vi "CAL_GCP_L.vi"(9 "출력 클러스터 2":T1, 10 "B_ACC":sgl, 11 "L_ROLL":sgl) -> (0 "L_Period":sgl, 1 "L_GCP":sgl, 2 "L_Ctrl_Start":bool, 3 "L_NUM":u32, 4 "L_Run_OK":bool)   [LabVIEW 2019]
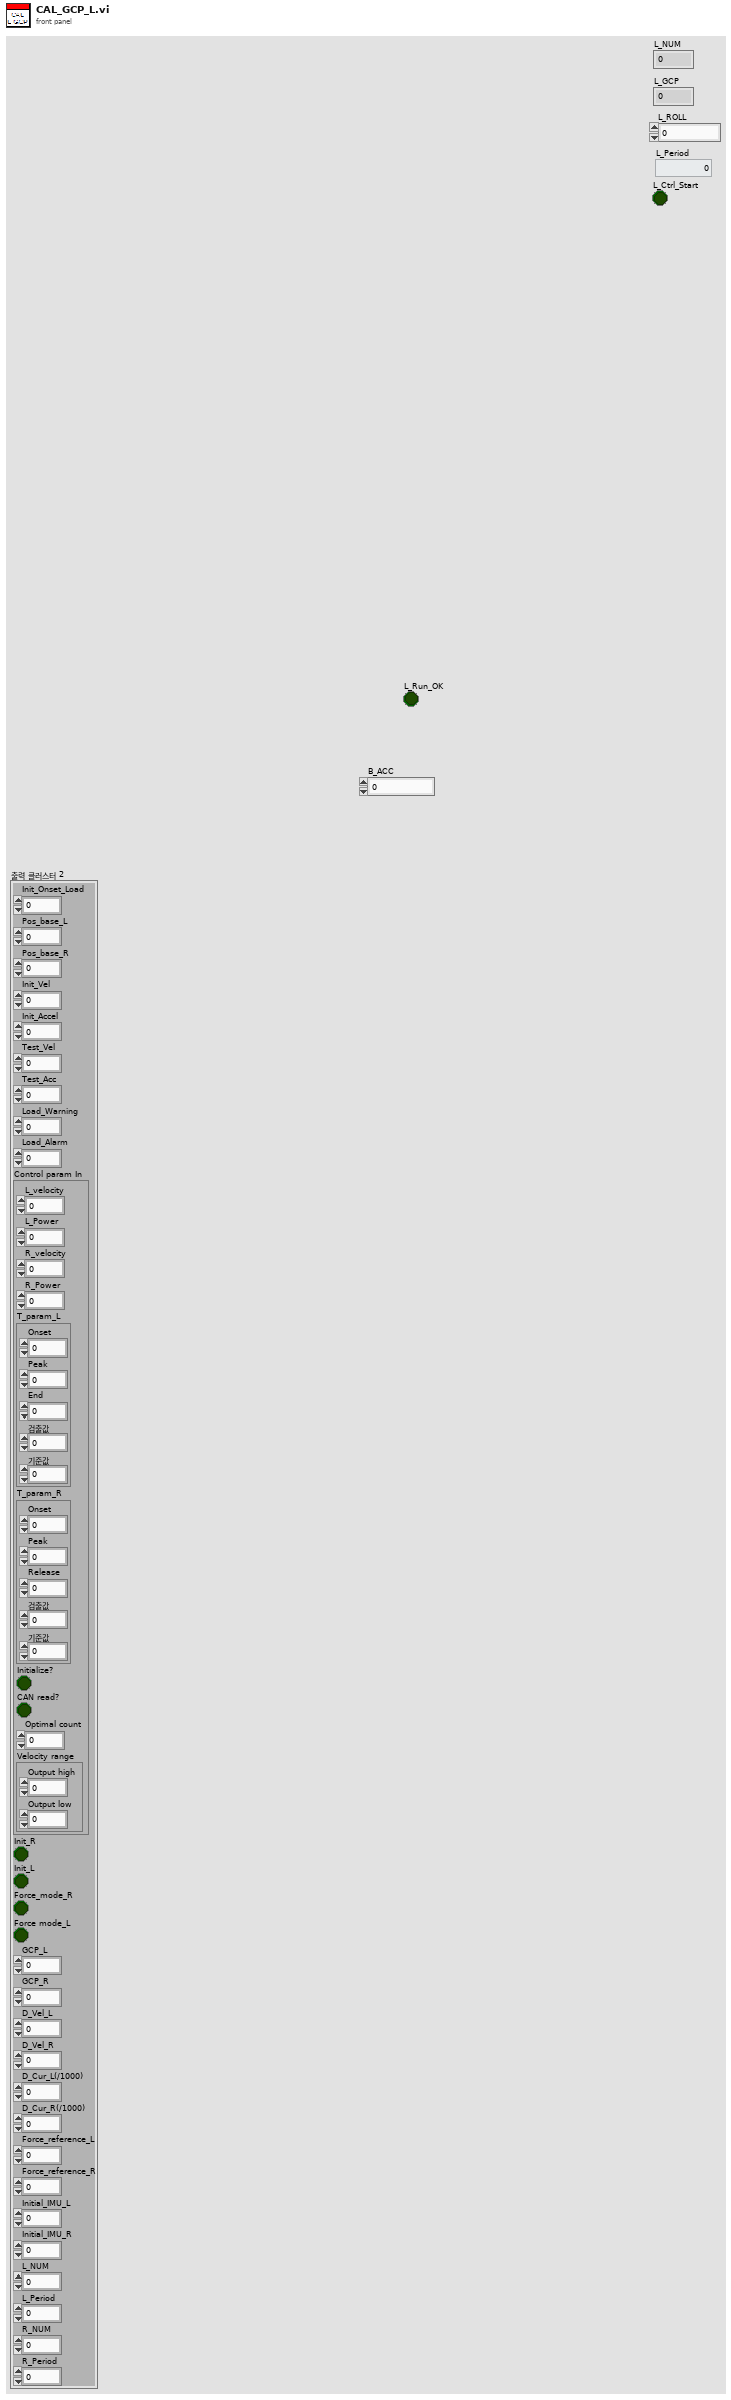
[diagram p1: front panel]
types:
  T1 = cluster{"Init_Onset_Load":sgl, "Pos_base_L":sgl, "Pos_base_R":sgl, "Init_Vel":i32, "Init_Accel":u32, "Test_Vel":i32, "Test_Acc":u32, "Load_Warning":sgl, "Load_Alarm":sgl, "Control param In":cluster{"L_velocity":u32, "L_Power":sgl, "R_velocity":u32, "R_Power":sgl, "T_param_L":cluster{"Onset":sgl, "Peak":sgl, "End":sgl, "검출값":sgl, "기준값":sgl}, "T_param_R":cluster{"Onset":sgl, "Peak":sgl, "Release":sgl, "검출값":sgl, "기준값":sgl}, "Initialize?":bool, "CAN read?":bool, "Optimal count":i32, "Velocity range":cluster{"Output high":dbl, "Output low":dbl}}, "Init_R":bool, "Init_L":bool, "Force_mode_R":bool, "Force mode_L":bool, "GCP_L":sgl, "GCP_R":sgl, "D_Vel_L":sgl, "D_Vel_R":sgl, "D_Cur_L(/1000)":sgl, "D_Cur_R(/1000)":sgl, "Force_reference_L":sgl, "Force_reference_R":sgl, "Initial_IMU_L":sgl, "Initial_IMU_R":sgl, "L_NUM":u32, "L_Period":i16, "R_NUM":u32, "R_Period":i16}
  T2 = enum16{"Init", "HF", "Cross", "HE", "Cross_E", "Init_F"}
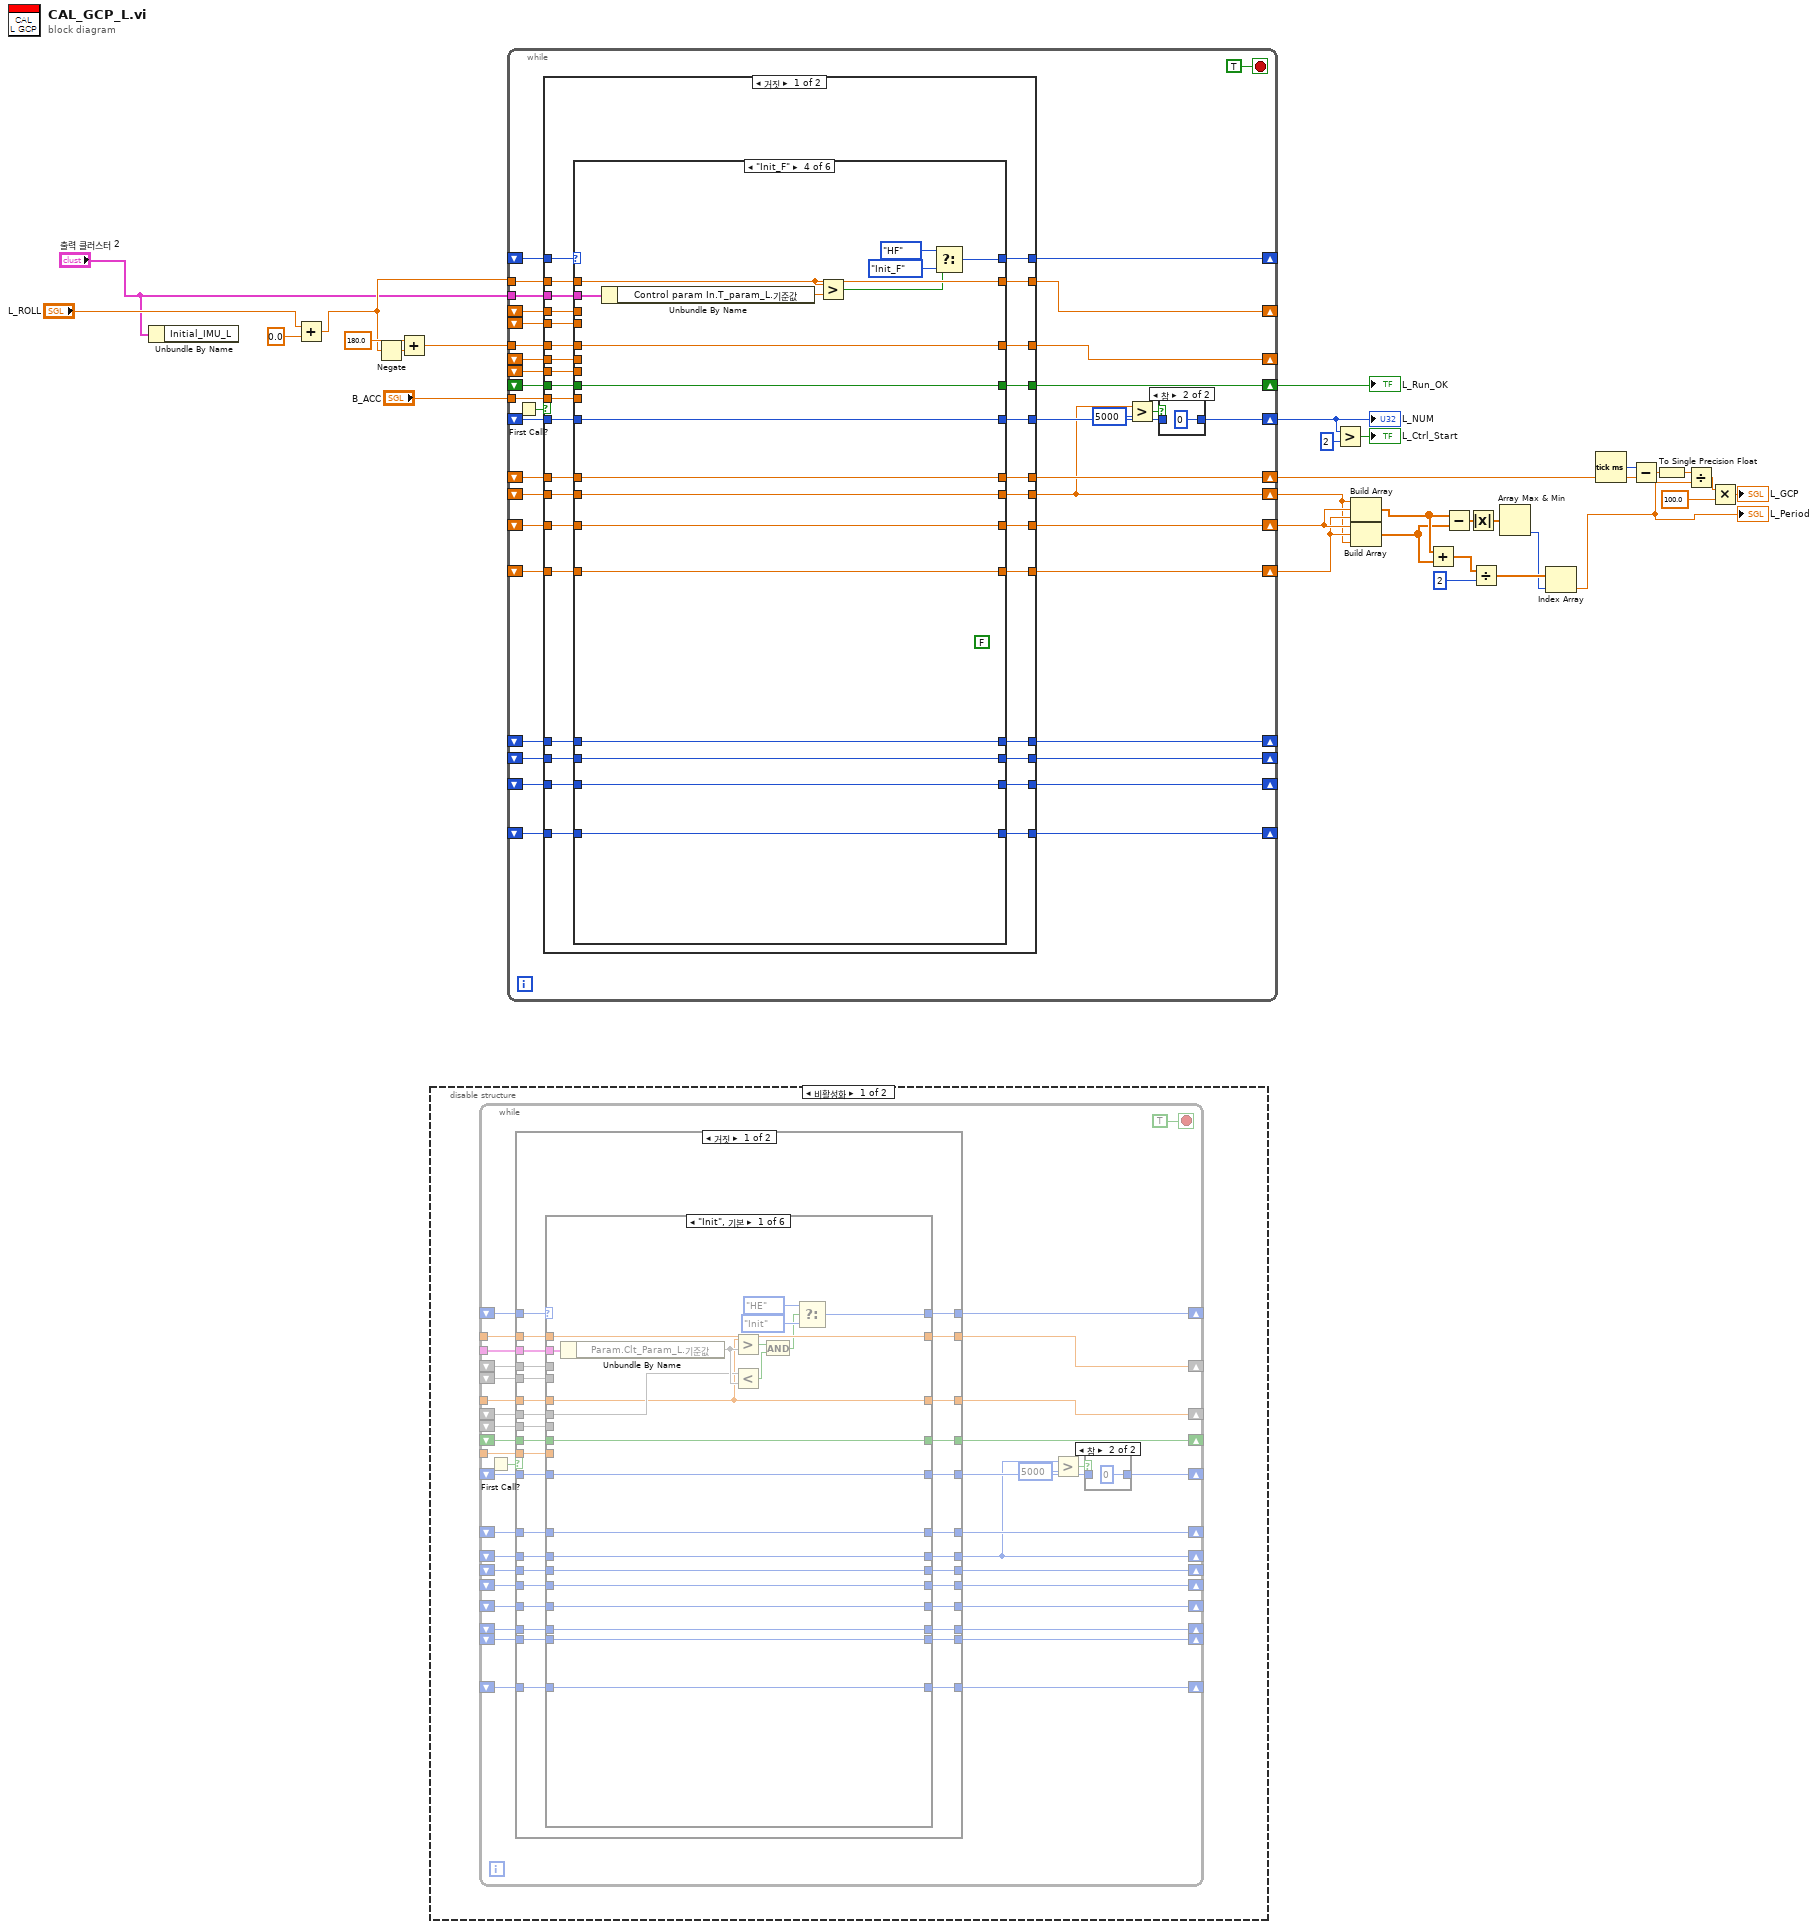
[diagram p0: block diagram]
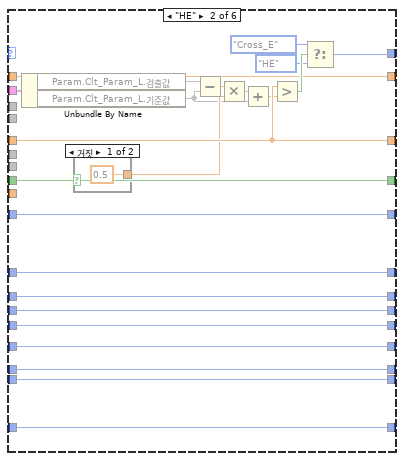
[diagram p2: hidden frame]
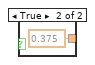
[diagram p3: hidden frame]
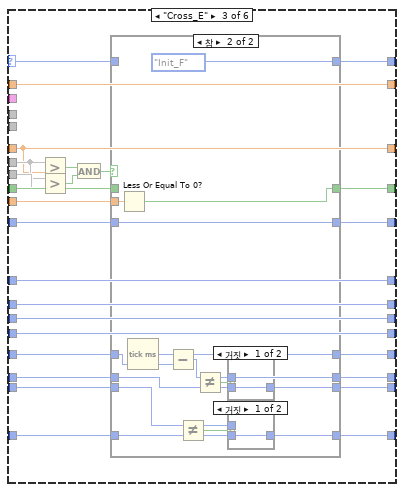
[diagram p4: hidden frame]
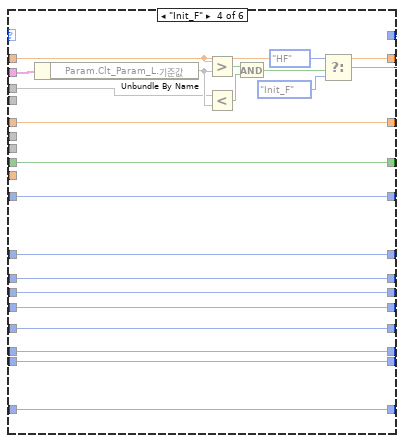
[diagram p8: hidden frame]
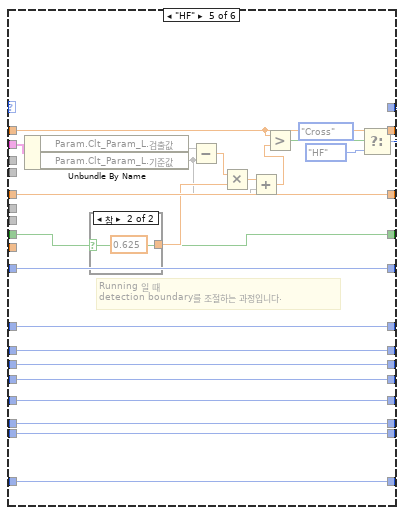
[diagram p9: hidden frame]
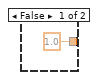
[diagram p10: hidden frame]
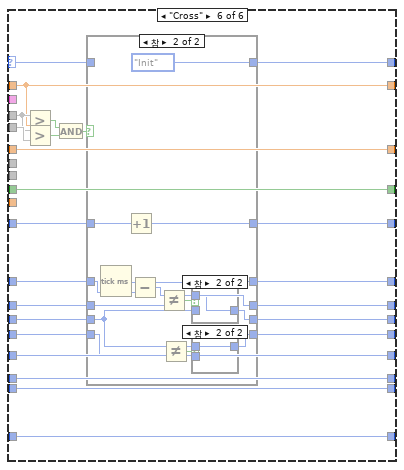
[diagram p11: hidden frame]
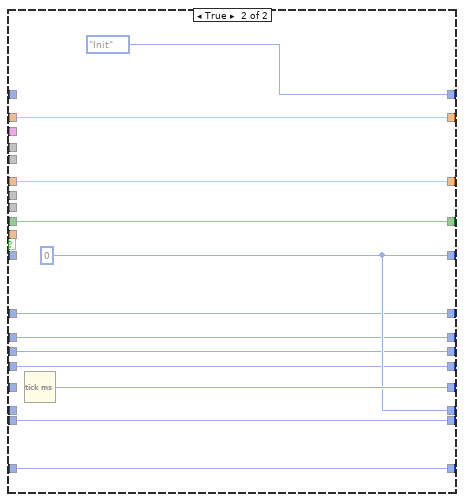
[diagram p15: hidden frame]
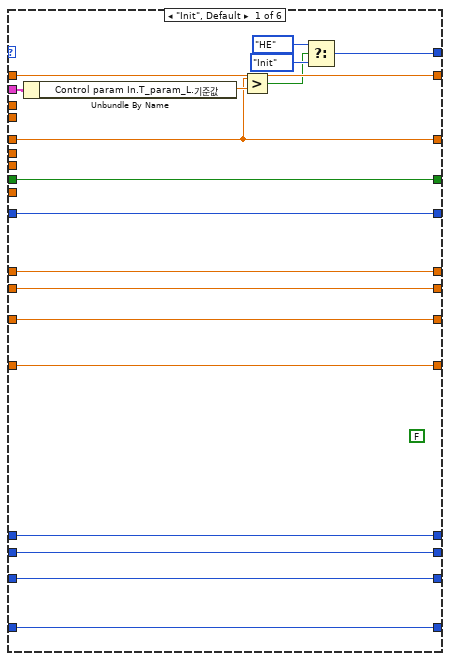
[diagram p18: hidden frame]
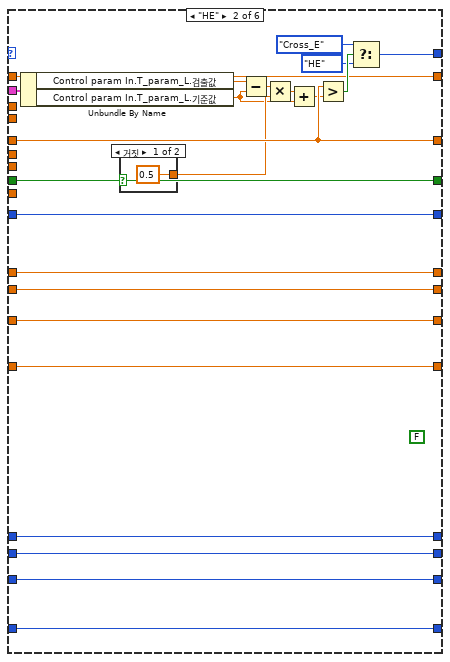
[diagram p19: hidden frame]
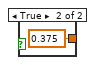
[diagram p20: hidden frame]
diagram:
  n1 = Unbundle By Name("출력 클러스터 2") -> ()  [unwired: 1 out]
  n2 = Add(x="L_ROLL", y=sgl 0.0) -> (x+y=w4:sgl)
  n3 = Negate(x=w4) -> (-x=w22:sgl)
  n4 = Add(x=sgl 180.0, y=w22) -> (x+y=w21:sgl)
  n5 = disable-structure shown="비활성화" {
    frame Disabled {
      n6 = while {
        tunnel: _ -> [w65]
        tunnel: _ -> [w62]
        shift-right: [w34] -> _
        shift-left: _ -> [w33]
        shift-right: [w66] -> _
        shift-left: _ -> [w61]
        shift-left: _ -> [w60]
        shift-right: [w57] -> _
        shift-left: _ -> [w64]
        shift-right: [w47] -> _
        shift-left: _ -> [w63]
        tunnel: _ -> [w55]
        shift-right: [w54] -> _
        shift-left: _ -> [w53]
        shift-left: _ -> [w52]
        shift-right: [w51] -> _
        shift-left: _ -> [w50]
        tunnel: _ -> [w49]
        shift-right: [w46] -> _
        shift-left: _ -> [w48]
        shift-right: [w39] -> _
        shift-left: _ -> [w38]
        shift-right: [w36] -> _
        shift-left: _ -> [w37]
        shift-right: [w45] -> _
        shift-left: _ -> [w44]
        shift-right: [w42] -> _
        shift-left: _ -> [w43]
        shift-right: [w41] -> _
        shift-left: _ -> [w40]
        shift-right: [w32] -> _
        shift-left: _ -> [w35]
        stop <- TRUE stop-if-true
        n7 = First Call?() -> (First Call?: T/F=w67:bool)
        n8 = case shown="거짓" w67 {
          tunnel: [w98 w302] -> w66
          tunnel: w65 -> [w99 w302]
          tunnel: w64 -> [w96 _]
          tunnel: [w97 w300] -> w56
          tunnel: [w94 w301] -> w47
          tunnel: [w93 w300] -> w46
          tunnel: w63 -> [w95 _]
          tunnel: w62 -> [w100 _]
          tunnel: w61 -> [w92 _]
          tunnel: w60 -> [w91 _]
          tunnel: w55 -> [w90 w299]
          tunnel: [w89 w299] -> w54
          tunnel: w53 -> [w88 _]
          tunnel: w52 -> [w87 _]
          tunnel: [w85 w298] -> w51
          tunnel: w50 -> [w86 w298]
          tunnel: w49 -> [w84 _]
          tunnel: w48 -> [w83 _]
          tunnel: [w82 w297] -> w45
          tunnel: w44 -> [w81 w297]
          tunnel: w43 -> [w80 w296]
          tunnel: [w79 w296] -> w42
          tunnel: [w78 w295] -> w41
          tunnel: w40 -> [w77 w295]
          tunnel: [w76 w294] -> w39
          tunnel: w38 -> [w75 w294]
          tunnel: w37 -> [w74 w293]
          tunnel: [w73 w293] -> w36
          tunnel: [w72 w292] -> w32
          tunnel: w35 -> [w71 w292]
          tunnel: [w69 T2."Init"] -> w34
          tunnel: w33 -> [w70 _]
          frame False {
            n9 = case shown="\"Init\", 기본" w70 {
              selector: w70 -> [_ _ w172 _ _ w267]
              tunnel: w100 -> [w118 w136 _ w212 w241 _]
              tunnel: w99 -> [w117 w143 w152 w209 w239 w260]
              tunnel: [w117 w143 w152 w209 w239 w260] -> w98
              tunnel: [w116 w142 w170 w206 w238 w262] -> w97
              tunnel: w96 -> [w116 w142 w171 w206 w238 w263]
              tunnel: w95 -> [w115 w141 w168 w205 w237 w255]
              tunnel: [w115 w141 w169 w205 w237 w255] -> w94
              tunnel: [w111 w140 w167 w204 w236 w258] -> w93
              tunnel: w92 -> [_ _ _ w211 _ w261]
              tunnel: w91 -> [_ _ _ _ _ w266]
              tunnel: w90 -> [w113 w135 w151 w208 w232 w252]
              tunnel: [w113 w135 w151 w208 w232 w252] -> w89
              tunnel: w88 -> [w114 _ w159 _ _ _]
              tunnel: w87 -> [_ _ w160 _ _ _]
              tunnel: w86 -> [w112 w126 w166 w207 w226 w251]
              tunnel: [w112 w126 w165 w207 w226 w251] -> w85
              tunnel: w84 -> [_ _ w164 _ _ _]
              tunnel: w83 -> [w111 w140 w158 w204 w236 w258]
              tunnel: [w110 w139 w157 w202 w235 w257] -> w82
              tunnel: w81 -> [w110 w139 w156 w202 w235 w257]
              tunnel: w80 -> [w109 w138 w155 w201 w234 w256]
              tunnel: [w109 w138 w154 w201 w234 w256] -> w79
              tunnel: [w108 w137 w153 w203 w233 w254] -> w78
              tunnel: w77 -> [w108 w137 w153 w203 w233 w253]
              tunnel: [w107 w134 w149 w199 w231 w250] -> w76
              tunnel: w75 -> [w107 w134 w149 w199 w231 w249]
              tunnel: w74 -> [w106 w133 w150 w198 w230 w248]
              tunnel: [w106 w133 w150 w198 w230 w247] -> w73
              tunnel: [w105 w125 w148 w200 w222 w246] -> w72
              tunnel: w71 -> [w105 w125 w148 w200 w222 w245]
              tunnel: [w104 w122 w147 w210 w219 w244] -> w69
              frame "Init", Default {
                n10 = Unbundle By Name(w118) -> ("Param.Clt_Param_L.기준값"=w119)
                n11 = Greater?(x=w113, y=w119) -> (0:w121:bool)
                n12 = Less?(x=w114, y=w119) -> (x < y?=w120:bool)
                n13 = And(x=w121, y=w120) -> (x .and. y?=w102:bool)
                n14 = Select(t=T2."HE", s=w102, f=T2."Init") -> (s? t:f=w104:T2)
              }
              frame "HE" {
                n15 = Unbundle By Name(w136) -> ("Param.Clt_Param_L.검출값"=w131, "Param.Clt_Param_L.기준값"=w128)
                n16 = case shown="거짓" w126 {
                  tunnel: [sgl 0.5 ("y") sgl 0.375 ("y")] -> w132
                  frame False {
                  }
                  frame True {
                  }
                }
                n17 = Subtract(x=w131, y=w128) -> (x-y=w130:dbl)
                n18 = Multiply(x=w130, y=w132) -> (x*y=w129:sgl)
                n19 = Add(x=w129, y=w128) -> (x+y=w127:sgl)
                n20 = Greater?(x=w135, y=w127) -> (0:w144:bool)
                n21 = Select(t=T2."Cross_E", s=w144, f=T2."HE") -> (s? t:f=w122:T2)
              }
              frame "Cross_E" {
                n22 = Greater?(x=w159, y=w151) -> (0:w162:bool)
                n23 = Greater?(x=w159, y=w160) -> (0:w163:bool)
                n24 = And(x=w162, y=w163) -> (x .and. y?=w161:bool)
                n25 = case shown="참" w161 {
                  tunnel: w172 -> [w177 _]
                  tunnel: [w177 T2."Init_F"] -> w147
                  tunnel: w171 -> [w178 w181]
                  tunnel: [w178 w181] -> w170
                  tunnel: w168 -> [w179 w193]
                  tunnel: [w175 w180] -> w167
                  tunnel: [w179 w192] -> w169
                  tunnel: w166 -> [w176 _]
                  tunnel: [w176 w188] -> w165
                  tunnel: w164 -> [_ w189]
                  tunnel: w158 -> [w175 w187]
                  tunnel: [w174 w186] -> w157
                  tunnel: w156 -> [w174 w185]
                  tunnel: w155 -> [w173 w184]
                  tunnel: [w173 w183] -> w154
                  frame False {
                  }
                  frame True {
                    n26 = Less Or Equal To 0?(x=w189) -> (x <= 0?=w188:bool)
                    n27 = Tick Count (ms)() -> (millisecond timer value=w192:u32)
                    n28 = Subtract(x=w192, y=w193) -> (x-y=w180:u32)
                    n29 = Not Equal?(x=w185, y=w184) -> (x != y?=w190:bool)
                    n30 = Not Equal?(x=w180, y=w187) -> (x != y?=w191:bool)
                    n31 = case shown="거짓" w191 {
                      tunnel: [w196 w197] -> w186
                      tunnel: w180 -> [_ w197]
                      tunnel: w187 -> [w196 _]
                      frame False {
                      }
                      frame True {
                      }
                    }
                    n32 = case shown="거짓" w190 {
                      tunnel: w185 -> [_ w195]
                      tunnel: w184 -> [w194 _]
                      tunnel: [w194 w195] -> w183
                      frame False {
                      }
                      frame True {
                      }
                    }
                  }
                }
              }
              frame "Init_F" {
                n33 = Unbundle By Name(w212) -> ("Param.Clt_Param_L.기준값"=w216)
                n34 = Greater?(x=w209, y=w216) -> (0:w218:bool)
                n35 = Less?(x=w211, y=w216) -> (x < y?=w217:bool)
                n36 = And(x=w218, y=w217) -> (x .and. y?=w214:bool)
                n37 = Select(t=T2."HF", s=w214, f=T2."Init_F") -> (s? t:f=w210:T2)
              }
              frame "HF" {
                # "Running 일 때 \ndetection boundary를 조절하는 과정입니다."
                n38 = Unbundle By Name(w241) -> ("Param.Clt_Param_L.검출값"=w229, "Param.Clt_Param_L.기준값"=w224)
                n39 = case shown="참" w226 {
                  tunnel: [sgl 1.0 ("y") sgl 0.625 ("y")] -> w227
                  frame False {
                  }
                  frame True {
                  }
                }
                n40 = Subtract(x=w229, y=w224) -> (x-y=w228:dbl)
                n41 = Multiply(x=w228, y=w227) -> (x*y=w225:sgl)
                n42 = Add(x=w225, y=w224) -> (x+y=w223:sgl)
                n43 = Greater?(x=w239, y=w223) -> (0:w240:bool)
                n44 = Select(t=T2."Cross", s=w240, f=T2."HF") -> (s? t:f=w219:T2)
              }
              frame "Cross" {
                n45 = Greater?(x=w261, y=w260) -> (0:w259:bool)
                n46 = Greater?(x=w261, y=w266) -> (0:w265:bool)
                n47 = And(x=w259, y=w265) -> (x .and. y?=w264:bool)
                n48 = case shown="참" w264 {
                  tunnel: w267 -> [w272 _]
                  tunnel: [w272 T2."Init"] -> w244
                  tunnel: w263 -> [w273 w276]
                  tunnel: [w273 w275] -> w262
                  tunnel: [w271 w283] -> w254
                  tunnel: w253 -> [w271 w284]
                  tunnel: [w270 w282] -> w250
                  tunnel: w249 -> [w270 w281]
                  tunnel: w248 -> [w269 w280]
                  tunnel: [w269 w279] -> w247
                  tunnel: [w268 w274] -> w246
                  tunnel: w245 -> [w268 w278]
                  frame False {
                  }
                  frame True {
                    n49 = Tick Count (ms)() -> (millisecond timer value=w283:u32)
                    n50 = Increment(x=w276) -> (x+1=w275:u32)
                    n51 = Subtract(x=w283, y=w284) -> (x-y=w274:u32)
                    n52 = Not Equal?(x=w274, y=w278) -> (x != y?=w286:bool)
                    n53 = Not Equal?(x=w281, y=w280) -> (x != y?=w285:bool)
                    n54 = case shown="참" w286 {
                      tunnel: w274 -> [_ w290]
                      tunnel: [w289 w290] -> w282
                      tunnel: w281 -> [w289 _]
                      frame False {
                      }
                      frame True {
                      }
                    }
                    n55 = case shown="참" w285 {
                      tunnel: w281 -> [_ w288]
                      tunnel: w280 -> [w287 _]
                      tunnel: [w287 w288] -> w279
                      frame False {
                      }
                      frame True {
                      }
                    }
                  }
                }
              }
            }
          }
          frame True {
            w300 = u32 0
            n56 = Tick Count (ms)() -> (millisecond timer value=w301:u32)
          }
        }
        n57 = Greater?(x=w32, y=u32 5000) -> (0:w58:bool)
        n58 = case shown="참" w58 {
          tunnel: [w303 u32 0] -> w57
          tunnel: w56 -> [w303 _]
          frame False {
          }
          frame True {
          }
        }
      }
    }
    frame Enabled {
    }
  }
  n59 = while {
    tunnel: w4 -> [w338]
    tunnel: "출력 클러스터 2" -> [w335]
    shift-right: [w307] -> _
    shift-left: _ -> [w306]
    shift-right: [w339] -> _
    shift-left: _ -> [w334]
    shift-left: _ -> [w333]
    shift-right: [w330] -> w18
    shift-left: _ -> [w337]
    shift-right: [w320] -> _
    shift-left: _ -> [w336]
    tunnel: w21 -> [w328]
    shift-right: [w327] -> _
    shift-left: _ -> [w326]
    shift-left: _ -> [w325]
    shift-right: [w324] -> w19
    shift-left: _ -> [w323]
    tunnel: "B_ACC" -> [w322]
    shift-right: [w319] -> _
    shift-left: _ -> [w321]
    shift-right: [w312] -> w16
    shift-left: _ -> [w311]
    shift-right: [w309] -> w15
    shift-left: _ -> [w310]
    shift-right: [w318] -> _
    shift-left: _ -> [w317]
    shift-right: [w315] -> _
    shift-left: _ -> [w316]
    shift-right: [w314] -> w17
    shift-left: _ -> [w313]
    shift-right: [w305] -> w14
    shift-left: _ -> [w308]
    stop <- TRUE stop-if-true
    n60 = First Call?() -> (First Call?: T/F=w340:bool)
    n61 = case shown="거짓" w340 {
      tunnel: [w371 w571] -> w339
      tunnel: w338 -> [w372 w571]
      tunnel: w337 -> [w369 _]
      tunnel: [w370 w570] -> w329
      tunnel: [w367 w561] -> w320
      tunnel: [w366 w570] -> w319
      tunnel: w336 -> [w368 _]
      tunnel: w335 -> [w373 _]
      tunnel: w334 -> [w365 _]
      tunnel: w333 -> [w364 _]
      tunnel: w328 -> [w363 w569]
      tunnel: [w362 w569] -> w327
      tunnel: w326 -> [w361 _]
      tunnel: w325 -> [w360 _]
      tunnel: [w358 w568] -> w324
      tunnel: w323 -> [w359 w568]
      tunnel: w322 -> [w357 _]
      tunnel: w321 -> [w356 _]
      tunnel: [w355 w567] -> w318
      tunnel: w317 -> [w354 w567]
      tunnel: w316 -> [w353 w566]
      tunnel: [w352 w566] -> w315
      tunnel: [w351 w561] -> w314
      tunnel: w313 -> [w350 _]
      tunnel: [w349 w565] -> w312
      tunnel: w311 -> [w348 w565]
      tunnel: w310 -> [w347 w564]
      tunnel: [w346 w564] -> w309
      tunnel: [w345 w563] -> w305
      tunnel: w308 -> [w344 w563]
      tunnel: [w342 T2."Init"] -> w307
      tunnel: w306 -> [w343 _]
      frame False {
        n62 = case shown="\"Init_F\"" w343 {
          selector: w343 -> [_ _ w442 _ _ w536]
          tunnel: w373 -> [w390 w406 _ w484 w510 _]
          tunnel: w372 -> [w389 w413 w422 w482 w508 w529]
          tunnel: [w389 w413 w422 w482 w508 w529] -> w371
          tunnel: [w388 w412 w440 w479 w507 w531] -> w370
          tunnel: w369 -> [w388 w412 w441 w479 w507 w532]
          tunnel: w368 -> [w387 w411 w438 w478 w506 w524]
          tunnel: [w387 w411 w439 w478 w506 w524] -> w367
          tunnel: [w384 w410 w437 w477 w505 w527] -> w366
          tunnel: w365 -> [_ _ _ _ _ w530]
          tunnel: w364 -> [_ _ _ _ _ w535]
          tunnel: w363 -> [w386 w405 w421 w481 w501 w521]
          tunnel: [w386 w405 w421 w481 w501 w521] -> w362
          tunnel: w361 -> [_ _ w429 _ _ _]
          tunnel: w360 -> [_ _ w430 _ _ _]
          tunnel: w359 -> [w385 w396 w436 w480 w495 w520]
          tunnel: [w385 w396 w435 w480 w495 w520] -> w358
          tunnel: w357 -> [_ _ w434 _ _ _]
          tunnel: w356 -> [w384 w410 w428 w477 w505 w527]
          tunnel: [w383 w409 w427 w475 w504 w526] -> w355
          tunnel: w354 -> [w383 w409 w426 w475 w504 w526]
          tunnel: w353 -> [w382 w408 w425 w474 w503 w525]
          tunnel: [w382 w408 w424 w474 w503 w525] -> w352
          tunnel: [w381 w407 w423 w476 w502 w523] -> w351
          tunnel: w350 -> [w381 w407 w423 w476 w502 w522]
          tunnel: [w380 w404 w419 w472 w500 w519] -> w349
          tunnel: w348 -> [w380 w404 w419 w472 w500 w518]
          tunnel: w347 -> [w379 w403 w420 w471 w499 w517]
          tunnel: [w379 w403 w420 w471 w499 w516] -> w346
          tunnel: [w378 w395 w418 w473 w491 w515] -> w345
          tunnel: w344 -> [w378 w395 w418 w473 w491 w514]
          tunnel: [w377 w392 w417 w483 w488 w513] -> w342
          frame "Init", Default {
            (unwired) FALSE
            n63 = Unbundle By Name(w390) -> ("Control param In.T_param_L.기준값"=w391:sgl)
            n64 = Greater?(x=w386, y=w391) -> (0:w374:bool)
            n65 = Select(t=T2."HE", s=w374, f=T2."Init") -> (s? t:f=w377:T2)
          }
          frame "HE" {
            (unwired) FALSE
            n66 = Unbundle By Name(w406) -> ("Control param In.T_param_L.검출값"=w401:sgl, "Control param In.T_param_L.기준값"=w398:sgl)
            n67 = case shown="거짓" w396 {
              tunnel: [sgl 0.5 ("y") sgl 0.375 ("y")] -> w402
              frame False {
              }
              frame True {
              }
            }
            n68 = Subtract(x=w401, y=w398) -> (x-y=w400:sgl)
            n69 = Multiply(x=w400, y=w402) -> (x*y=w399:sgl)
            n70 = Add(x=w399, y=w398) -> (x+y=w397:sgl)
            n71 = Greater?(x=w405, y=w397) -> (0:w414:bool)
            n72 = Select(t=T2."Cross_E", s=w414, f=T2."HE") -> (s? t:f=w392:T2)
          }
          frame "Cross_E" {
            (unwired) FALSE
            n73 = Greater?(x=w429, y=w421) -> (0:w432:bool)
            n74 = Greater Or Equal?(x=w429, y=w430) -> (x >= y?=w433:bool)
            n75 = And(x=w432, y=w433) -> (x .and. y?=w431:bool)
            n76 = case shown="참" w431 {
              tunnel: w442 -> [w447 _]
              tunnel: [w447 T2."Init_F"] -> w417
              tunnel: w441 -> [w448 w456]
              tunnel: [w448 w456] -> w440
              tunnel: w438 -> [w449 w465]
              tunnel: [w445 w455] -> w437
              tunnel: [w449 w464] -> w439
              tunnel: w436 -> [w446 _]
              tunnel: [w446 w461] -> w435
              tunnel: w434 -> [_ w452]
              tunnel: w428 -> [w445 w454]
              tunnel: [w444 w460] -> w427
              tunnel: w426 -> [w444 w453]
              tunnel: w425 -> [w443 w459]
              tunnel: [w443 w458] -> w424
              frame False {
              }
              frame True {
                n77 = Tick Count (ms)() -> (millisecond timer value=w464:u32)
                n78 = Subtract(x=w464, y=w465) -> (x-y=w455:u32)
                n79 = Add(x=w452, y=9.8) -> (x+y=w450:dbl)
                n80 = Not Equal?(x=w453, y=w459) -> (x != y?=w462:bool)
                n81 = Not Equal?(x=w454, y=w453) -> (x != y?=w463:bool)
                n82 = Greater Or Equal To 0?(x=w450) -> (x >= 0?=w461:bool)
                n83 = case shown="거짓" w463 {
                  tunnel: [w468 w469] -> w460
                  tunnel: w454 -> [_ w469]
                  tunnel: w453 -> [w468 _]
                  frame False {
                  }
                  frame True {
                  }
                }
                n84 = case shown="거짓" w462 {
                  tunnel: w453 -> [_ w467]
                  tunnel: w459 -> [w466 _]
                  tunnel: [w466 w467] -> w458
                  frame False {
                  }
                  frame True {
                  }
                }
              }
            }
          }
          frame "Init_F" {
            (unwired) FALSE
            n85 = Unbundle By Name(w484) -> ("Control param In.T_param_L.기준값"=w487:sgl)
            n86 = Greater?(x=w482, y=w487) -> (0:w470:bool)
            n87 = Select(t=T2."HF", s=w470, f=T2."Init_F") -> (s? t:f=w483:T2)
          }
          frame "HF" {
            (unwired) FALSE
            # "Running 일 때 \ndetection boundary를 조절하는 과정입니다."
            n88 = Unbundle By Name(w510) -> ("Control param In.T_param_L.검출값"=w498:sgl, "Control param In.T_param_L.기준값"=w493:sgl)
            n89 = case shown="참" w495 {
              tunnel: [sgl 1.0 ("y") sgl 0.625 ("y")] -> w496
              frame False {
              }
              frame True {
              }
            }
            n90 = Subtract(x=w498, y=w493) -> (x-y=w497:sgl)
            n91 = Multiply(x=w497, y=w496) -> (x*y=w494:sgl)
            n92 = Add(x=w494, y=w493) -> (x+y=w492:sgl)
            n93 = Greater?(x=w508, y=w492) -> (0:w509:bool)
            n94 = Select(t=T2."Cross", s=w509, f=T2."HF") -> (s? t:f=w488:T2)
          }
          frame "Cross" {
            n95 = Greater?(x=w530, y=w529) -> (0:w528:bool)
            n96 = Greater Or Equal?(x=w530, y=w535) -> (x >= y?=w534:bool)
            n97 = And(x=w528, y=w534) -> (x .and. y?=w533:bool)
            n98 = case shown="참" w533 {
              tunnel: w536 -> [w541 _]
              tunnel: [w541 T2."Init"] -> w513
              tunnel: w532 -> [w542 w549]
              tunnel: [w542 w548] -> w531
              tunnel: [w540 w543] -> w523
              tunnel: w522 -> [w540 w554]
              tunnel: [w539 w553] -> w519
              tunnel: w518 -> [w539 w545]
              tunnel: w517 -> [w538 w552]
              tunnel: [w538 w551] -> w516
              tunnel: [w537 w547] -> w515
              tunnel: w514 -> [w537 w546]
              frame False {
              }
              frame True {
                n99 = call "Tick 카운트"() -> ("Tick Count(mSec)"=w544:u32)
                n100 = Increment(x=w549) -> (x+1=w548:u32)
                n101 = To Single Precision Float(number=w544) -> (single precision float=w543:sgl)
                n102 = Subtract(x=w543, y=w554) -> (x-y=w547:sgl)
                n103 = Not Equal?(x=w546, y=w545) -> (x != y?=w556:bool)
                n104 = Not Equal?(x=w545, y=w552) -> (x != y?=w555:bool)
                n105 = case shown="참" w556 {
                  tunnel: w546 -> [_ w560]
                  tunnel: [w559 w560] -> w553
                  tunnel: w545 -> [w559 _]
                  frame False {
                  }
                  frame True {
                  }
                }
                n106 = case shown="참" w555 {
                  tunnel: w545 -> [_ w558]
                  tunnel: w552 -> [w557 _]
                  tunnel: [w557 w558] -> w551
                  frame False {
                  }
                  frame True {
                  }
                }
              }
            }
          }
        }
      }
      frame True {
        (unwired) FALSE
        w570 = u32 0
        n107 = Tick Count (ms)() -> (millisecond timer value=w561:u32)
      }
    }
    n108 = Greater?(x=w305, y=u32 5000) -> (0:w331:bool)
    n109 = case shown="참" w331 {
      tunnel: [w572 u32 0] -> w330
      tunnel: w329 -> [w572 _]
      frame False {
      }
      frame True {
      }
    }
  }
  "L_NUM" <- w18
  "L_Run_OK" <- w19
  n110 = Greater?(x=w18, y=u32 2) -> (0:→"L_Ctrl_Start":bool)
  n111 = Build Array(w14, w16, w15) -> (w7:sgl[])
  n112 = Build Array(w16, w15, w14) -> (w6:sgl[])
  n113 = Add(x=w7, y=w6) -> (x+y=w11:sgl[])
  n114 = Subtract ("빼기")(x=w7, y=w6) -> (x-y=w13:sgl[])
  n115 = Absolute Value(x=w13) -> (abs(x)=w12:sgl[])
  n116 = Divide ("나누기")(x=w11, y=2) -> (x/y=w9:sgl[])
  n117 = Array Max & Min(array=w12) -> (min index (indices)=w8:i32)  [unwired: 3 out]
  n118 = Index Array(array=w9, index=w8) -> (element=w5:sgl)
  "L_Period" <- w5
  n119 = Tick Count (ms)() -> (millisecond timer value=w27:u32)
  n120 = Subtract(x=w27, y=w17) -> (x-y=w26:sgl)
  n121 = To Single Precision Float(number=w26) -> (single precision float=w24:sgl)
  n122 = Divide(x=w24, y=w5) -> (x/y=w29:sgl)
  n123 = Multiply(x=w29, y=sgl 100.0) -> (x*y=→"L_GCP":sgl)
